vi "read_signal.vi"(8 "error in (no error)":errorcluster, 11 "Dust Event ID":i32) -> (0 "error out":errorcluster, 3 "Signal Array":T1[](array[typedef]))   [LabVIEW 2013]
uses:
  Public API/Post_Signal.ctl
  Controls/Role ID.ctl
  Controls/Hardware ID.ctl
  <vilib>/addons/h5labview/H5F_mode.ctl
  <vilib>/addons/h5labview/polymorph/H5A_read_var.vi
  <vilib>/addons/h5labview/H5File.lvlib
  <vilib>/addons/h5labview/H5GroupObject.lvlib
  <vilib>/addons/h5labview/H5Attrib.lvlib
panel:
  out "size(s)":i32
  out "names":string[](array[string])
  # "Signal"
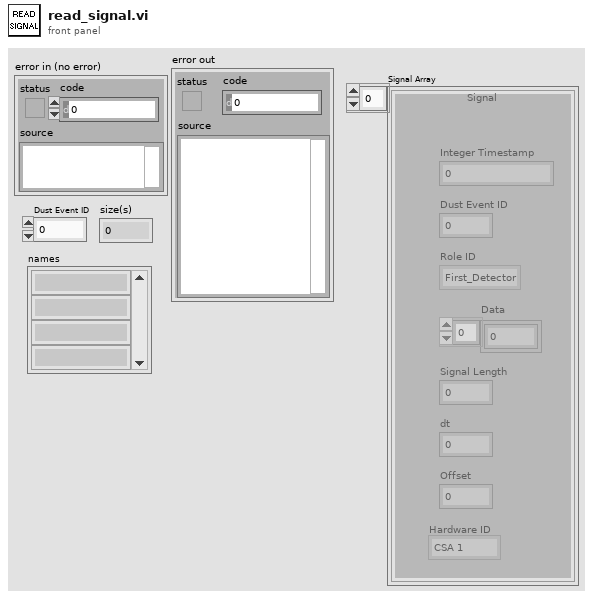
[diagram p1: front panel]
types:
  T1 = typedef "Post_Signal.ctl" = cluster{"Integer Timestamp":i64, "Dust Event ID":i64, "Role ID":T2, "Data":sgl[], "Signal Length":i32, "dt":sgl, "Offset":dbl, "Hardware ID":T3}
  T2 = typedef "Role ID.ctl" = enum16{"First_Detector", "Second_Detector", "Third_Detector", "LeCroy_CH1", "LeCroy_CH2", "LeCroy_CH3", "LeCroy_CH4", "PSU"}
  T3 = typedef "Hardware ID.ctl" = enum16{"Unknown", "CSA 1", "CSA 2", "CSA 3", "CSA 4", "CSA 5", "CSA 6"}
  T4 = typedef "H5File.lvlib/H5F_mode.ctl" = enum16{"read-only", "read-write", "overwrite", "create new", "open or create"}
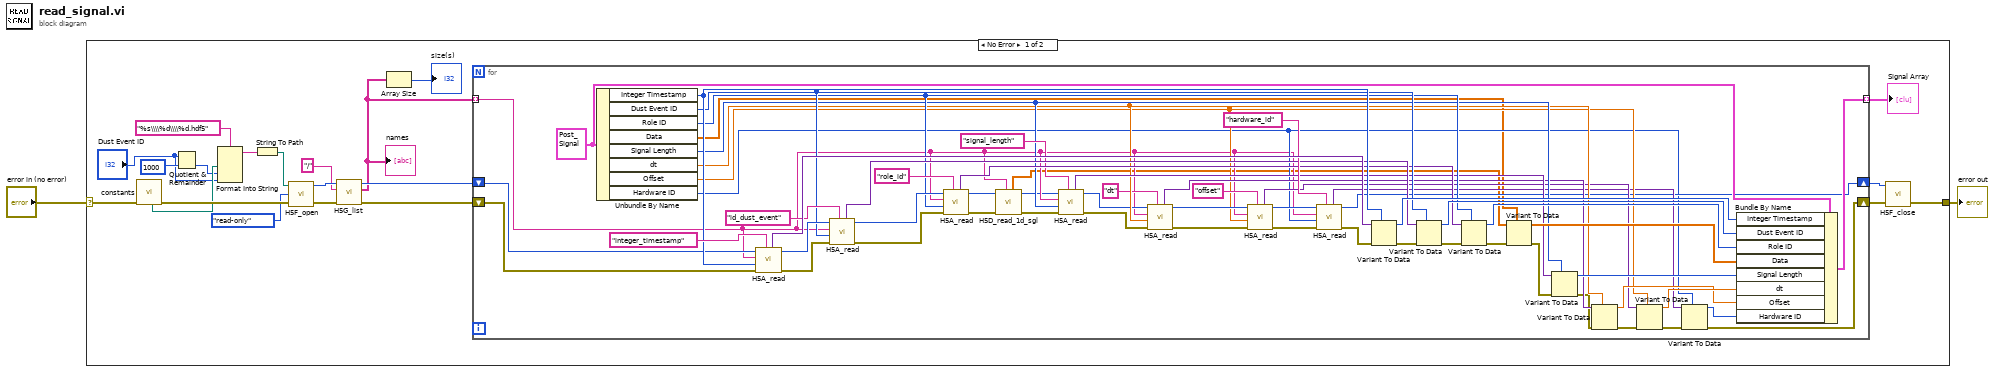
[diagram p0: block diagram]
diagram:
  n1 = case shown="No Error" "error in (no error)" {
    selector: "error in (no error)" -> [w21 w84]
    tunnel: [w23 w84] -> w2
    frame No Error {
      n2 = call "constants.vi"("error in (no error)"=w21) -> ("error out"=w22:errorcluster, "Waveforms path"=w6:path)  [unwired: 5 in, 4 out]
      n3 = Quotient & Remainder(x="Dust Event ID", y=1000) -> (floor(x/y)=w5:i32)  [unwired: 1 out]
      n4 = Format Into String(format string="%s\\\\%d\\\\%d.hdf5", w6, w5, "Dust Event ID") -> (resulting string=w3:string)  [unwired: 2 in, 1 out]
      n5 = String To Path(string=w3) -> (path=w20:path)
      n6 = call <vilib>:"H5F_open.vi"("error in (no error)"=w22, "mode"=H5F_mode."read-only", "path"=w20) -> ("error out"=w17:errorcluster, "ref"=w18:i32)  [unwired: 1 in]
      n7 = call <vilib>:"H5G_list.vi"("error in (no error)"=w17, "group"="/", "ref"=w18) -> ("error out"=w15:errorcluster, "names"=w9:string[], "ref out"=w14:i32)  [unwired: 1 in, 1 out]
      "names" <- w9
      n8 = Array Size(array=w9) -> (size(s)=→"size(s)":i32)
      n9 = for {
        shift-right: [w31] -> w13
        shift-left: w15 -> [w74]
        shift-right: [w36] -> w12
        shift-left: w14 -> [w75]
        tunnel: [w81] -> w11 mode=indexing
        tunnel: w9 -> [w28] mode=indexing
        w83 = T1 {"Integer Timestamp"=0, "Dust Event ID"=0, "Role ID"=enum."First_Detector", "Data"=[], "Signal Length"=0, "dt"=0.0, "Offset"=0.0, "Hardware ID"=enum."CSA 1"} ("Post_Signal 2")
        n10 = Unbundle By Name(w83) -> ("Integer Timestamp"=w79:i64, "Dust Event ID"=w69:i64, "Role ID"=w62:T2, "Data"=w30:sgl[], "Signal Length"=w56:i32, "dt"=w52:sgl, "Offset"=w42:dbl, "Hardware ID"=w33:T3)
        n11 = call-poly <vilib>:"H5A_read.vi"("attrib_name"="integer_timestamp", "error in (no error)"=w74, "default"=w79, "obj_name"=w28, "ref"=w75) -> ("error out"=w71:errorcluster, "ref out"=w73:i32, "value"=w78:variant)  [unwired: 2 in]
        n12 = call-poly <vilib>:"H5A_read.vi"("attrib_name"="id_dust_event", "error in (no error)"=w71, "default"=w69, "obj_name"=w28, "ref"=w73) -> ("error out"=w66:errorcluster, "ref out"=w65:i32, "value"=w70:variant)  [unwired: 2 in]
        n13 = call-poly <vilib>:"H5A_read.vi"("attrib_name"="role_id", "error in (no error)"=w66, "default"=w62, "obj_name"=w28, "ref"=w65) -> ("error out"=w25:errorcluster, "ref out"=w29:i32, "value"=w63:variant)  [unwired: 2 in]
        n14 = call "H5D_read_1d_sgl.vi"("name"=w28, "error in (no error)"=w25, "ref"=w29) -> ("error out"=w24:errorcluster, "ref out"=w27:i32, "data"=w26:sgl[])  [unwired: 4 in]
        n15 = call-poly <vilib>:"H5A_read.vi"("attrib_name"="signal_length", "error in (no error)"=w24, "default"=w56, "obj_name"=w28, "ref"=w27) -> ("error out"=w48:errorcluster, "ref out"=w49:i32, "value"=w57:variant)  [unwired: 2 in]
        n16 = call-poly <vilib>:"H5A_read.vi"("attrib_name"="dt", "error in (no error)"=w48, "default"=w52, "obj_name"=w28, "ref"=w49) -> ("error out"=w45:errorcluster, "ref out"=w46:i32, "value"=w53:variant)  [unwired: 2 in]
        n17 = call-poly <vilib>:"H5A_read.vi"("attrib_name"="offset", "error in (no error)"=w45, "default"=w42, "obj_name"=w28, "ref"=w46) -> ("error out"=w38:errorcluster, "ref out"=w39:i32, "value"=w43:variant)  [unwired: 2 in]
        n18 = call-poly <vilib>:"H5A_read.vi"("attrib_name"="hardware_id", "error in (no error)"=w38, "default"=w33, "obj_name"=w28, "ref"=w39) -> ("error out"=w35:errorcluster, "ref out"=w36:i32, "value"=w37:variant)  [unwired: 2 in]
        n19 = Variant To Data(error in=w35, type=w79, Variant=w78) -> (data=w77:i64, error out=w67:errorcluster)
        n20 = Variant To Data(error in=w67, type=w69, Variant=w70) -> (data=w68:i64, error out=w60:errorcluster)
        n21 = Variant To Data(error in=w60, type=w62, Variant=w63) -> (data=w61:T2, error out=w59:errorcluster)
        n22 = Variant To Data(error in=w59, type=w30, Variant=w26) -> (data=w82:sgl[], error out=w55:errorcluster)
        n23 = Variant To Data(error in=w55, type=w56, Variant=w57) -> (data=w54:i32, error out=w50:errorcluster)
        n24 = Variant To Data(error in=w50, type=w52, Variant=w53) -> (data=w51:sgl, error out=w40:errorcluster)
        n25 = Variant To Data(error in=w40, type=w42, Variant=w43) -> (data=w41:dbl, error out=w34:errorcluster)
        n26 = Variant To Data(error in=w34, type=w33, Variant=w37) -> (data=w32:T3, error out=w31:errorcluster)
        n27 = Bundle By Name(cluster=w83, "Integer Timestamp"=w77, "Dust Event ID"=w68, "Role ID"=w61, "Data"=w82, "Signal Length"=w54, "dt"=w51, "Offset"=w41, "Hardware ID"=w32) -> (w81:T1)
      }
      "Signal Array" <- w11
      n28 = call <vilib>:"H5F_close.vi"("error in (no error)"=w13, "ref"=w12) -> ("error out"=w23:errorcluster)  [unwired: 3 in]
    }
    frame Error {
    }
  }
  "error out" <- w2
